vi "FdxCmdIrigTimeControlCvi.vi"(8 "error in":errorcluster, 9 "Irig In":T2 {"Control" items=["FDX_IRIG_READ", "FDX_IRIG_WRITE", "FDX_IRIG_EXTERN", "FDX_IRIG_INTERN"]}, 11 "InstrumentHandle_board in":u32) -> (0 "error out":errorcluster, 1 "Irig Out":T1, 3 "InstrumentHandle_board out":u32)   [LabVIEW 2020, in "AIM664LV.lvlib"]
doc: "This function is used to read or set the on-board IRIG timecode encoder and also to select the IRIG source. There is a board internal IRIG time source, but it is also possible to synchronize the time coding to an external IRIG source."
uses:
  AIM664LV.lvlib
  AFDX_LibraryAdmin/FdxGlobalDllPath.vi
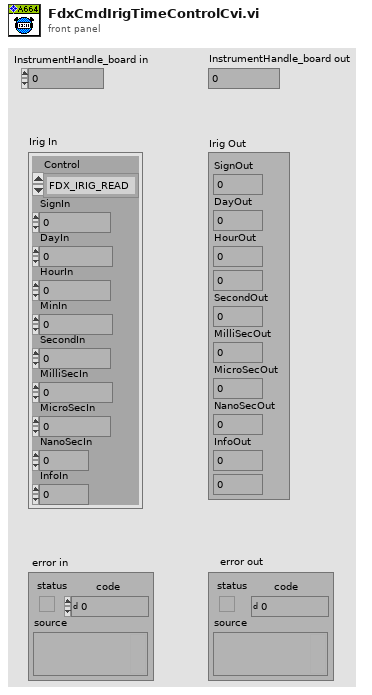
[diagram p1: front panel]
types:
  T1 = cluster{"SignOut":i32, "DayOut":u32, "HourOut":u32, "MinOut":u32, "SecondOut":u32, "MilliSecOut":u32, "MicroSecOut":u32, "NanoSecOut":u32, "InfoOut":u32, "Mode":u32}
  T2 = cluster{"Control":u32, "SignIn":i32, "DayIn":u32, "HourIn":u32, "MinIn":u32, "SecondIn":u32, "MilliSecIn":u32, "MicroSecIn":u32, "NanoSecIn":u32, "InfoIn":u32}
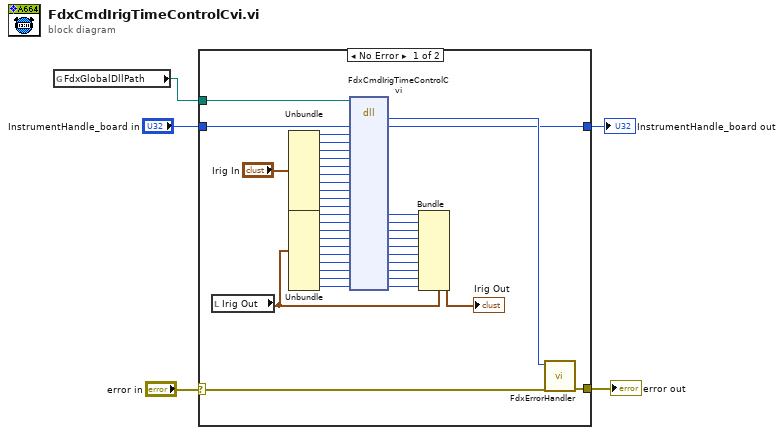
[diagram p0: block diagram]
diagram:
  n1 = global read "FdxGlobalDllPath.vi" "FdxGlobalDllPath"() -> (w3:path)
  n2 = case shown="No Error" "error in" {
    selector: "error in" -> [w42 w45]
    tunnel: [w43 w45] -> w5
    tunnel: w3 -> [w8 _]
    tunnel: [w7 w44] -> w2
    tunnel: "InstrumentHandle_board in" -> [w6 w44]
    frame No Error {
      n3 = local read "Irig Out"() -> (w9:T1)
      n4 = Unbundle("Irig In") -> ("Control"=w38:u32, "SignIn"=w37:i32, "DayIn"=w36:u32, "HourIn"=w35:u32, "MinIn"=w34:u32, "SecondIn"=w33:u32, "MilliSecIn"=w25:u32, "MicroSecIn"=w24:u32, "NanoSecIn"=w32:u32)  [unwired: 1 out]
      n5 = Unbundle(w9) -> ("SignOut"=w19:i32, "DayOut"=w18:u32, "HourOut"=w17:u32, "MinOut"=w16:u32, "SecondOut"=w15:u32, "MilliSecOut"=w14:u32, "MicroSecOut"=w13:u32, "NanoSecOut"=w12:u32, "InfoOut"=w11:u32, "Mode"=w10:u32)
      n6 = dll-call lib="aim_fdx.19.dll" fn="FdxCmdIrigTimeControlCvi"(path in=w8, "InstrumentHandle"=w6, "Control"=w38, "SignIn"=w37, "DayIn"=w36, "HourIn"=w35, "MinIn"=w34, "SecondIn"=w33, "MilliSecIn"=w25, "MicroSecIn"=w24, "NanoSecIn"=w32, "InfoIn"=w25, "SignOut"=w19, "DayOut"=w18, "HourOut"=w17, "MinOut"=w16, "SecondOut"=w15, "MilliSecOut"=w14, "MicroSecOut"=w13, "NanoSecOut"=w12, "InfoOut"=w11, "Mode"=w10) -> ("status"=w41:i32, "InstrumentHandle"=w7:u32, "SignOut"=w31:i32, "DayOut"=w30:u32, "HourOut"=w29:u32, "MinOut"=w28:u32, "SecondOut"=w27:u32, "MilliSecOut"=w26:u32, "MicroSecOut"=w23:u32, "NanoSecOut"=w22:u32, "InfoOut"=w21:u32, "Mode"=w20:u32)  [unwired: 12 in, 2 out]
      n7 = Bundle(cluster=w9, "SignOut"=w31, "DayOut"=w30, "HourOut"=w29, "MinOut"=w28, "SecondOut"=w27, "MilliSecOut"=w26, "MicroSecOut"=w23, "NanoSecOut"=w22, "InfoOut"=w21, "Mode"=w20) -> (→"Irig Out":T1)
      n8 = call "FdxErrorHandler.vi"("error in"=w42, "AIM Error"=w41) -> ("error out"=w43:errorcluster)  [unwired: 9 in]
    }
    frame Error {
    }
  }
  "error out" <- w5
  "InstrumentHandle_board out" <- w2
